vi "IPS Read Field Sweep Rate.vi"(0 "VISA resource name":refnum<visa-resource-name>="COM3", 1 "Error In":errorcluster={"status"=FALSE, "code"=1073676294, "source"="VISA Read in Prologix USB GPIB Command.vi"}) -> (2 "VISA resource name":refnum<visa-resource-name>="GPIB1::25::INSTR", 3 "Field Sweep Rate (T/min)":dbl, 4 "Error Out":errorcluster={"status"=FALSE, "code"=1073676294, "source"="VISA Read in Prologix_GPIB_Sample.vi"})   [LabVIEW 2013]
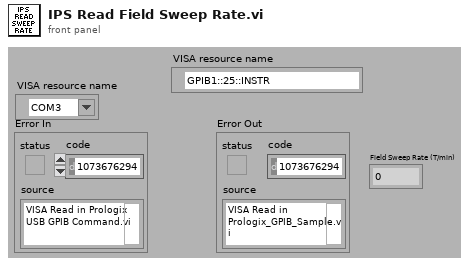
[diagram p1: front panel]
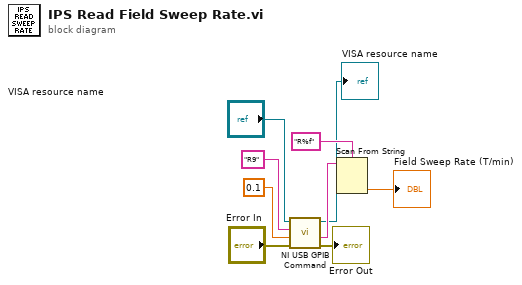
[diagram p0: block diagram]
diagram:
  n1 = call "NI USB GPIB Command.vi"("Error In"="Error In", "Wait for instrument to respond (s)"=0.1, "String to Send"="R9", "VISA resource name (COM Port of Prologix Device)"="VISA resource name") -> ("Error Out"=→"Error Out":errorcluster, "Return String from Device (Not all commands return a String)"=w4:string, "VISA resource name (COM Port of Prologix Device) 2"=→"VISA resource name":refnum<visa-resource-name>)  [unwired: 1 out]
  n2 = Scan From String(format string="R%f", input string=w4) -> (output 1=→"Field Sweep Rate (T/min)":dbl)  [unwired: 2 in, 4 out]
